vi "loadHTTemperature.vi"(8 "error in (no error)":errorcluster, 9 "Entity":string="QAMT03", 11 "file (use dialog)":path=path "C:/temp/ht/Temperature/temperatureLog.txt") -> (0 "error out":errorcluster)   [LabVIEW 2012]
uses:
  <vilib>/addons/database/Connection.llb/DB Tools Open Connec (Path).vi
  <vilib>/addons/database/Connection.llb/Conn Execute.vi
  <vilib>/addons/database/Recordset.llb/Rec Fetch Integer Data (R).vi
  <vilib>/addons/database/Recordset.llb/Rec Destroy - Connection.vi
  <vilib>/addons/database/NI_Database_API.lvlib
panel:
  in  "Cluster":T1
  out "before substring 2":string
  out "before substring":string
  out "date/time string":string
  out "text":string
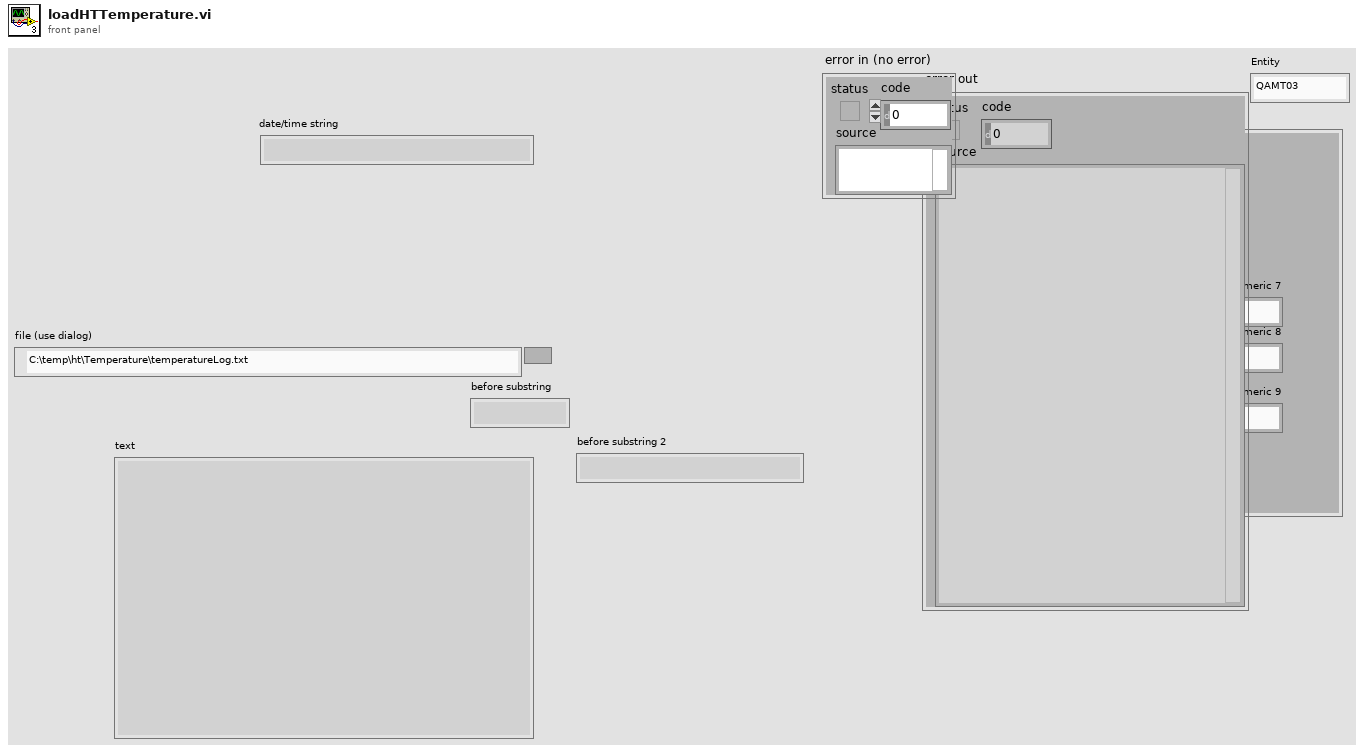
[diagram p1: front panel]
types:
  T1 = cluster{"Entity":string, "Time":string, "Numeric":dbl, "Numeric 2":dbl, "Numeric 3":dbl, "Numeric 4":dbl, "Numeric 5":dbl, "Numeric 6":dbl, "Numeric 7":dbl, "Numeric 8":dbl, "Numeric 9":dbl}
  T2 = typedef "NI_Database_API.lvlib/Conn ObjectReference.ctl" = refnum<k1>
  T3 = typedef "NI_Database_API.lvlib/Rec ObjectReference.ctl" = refnum<k1>
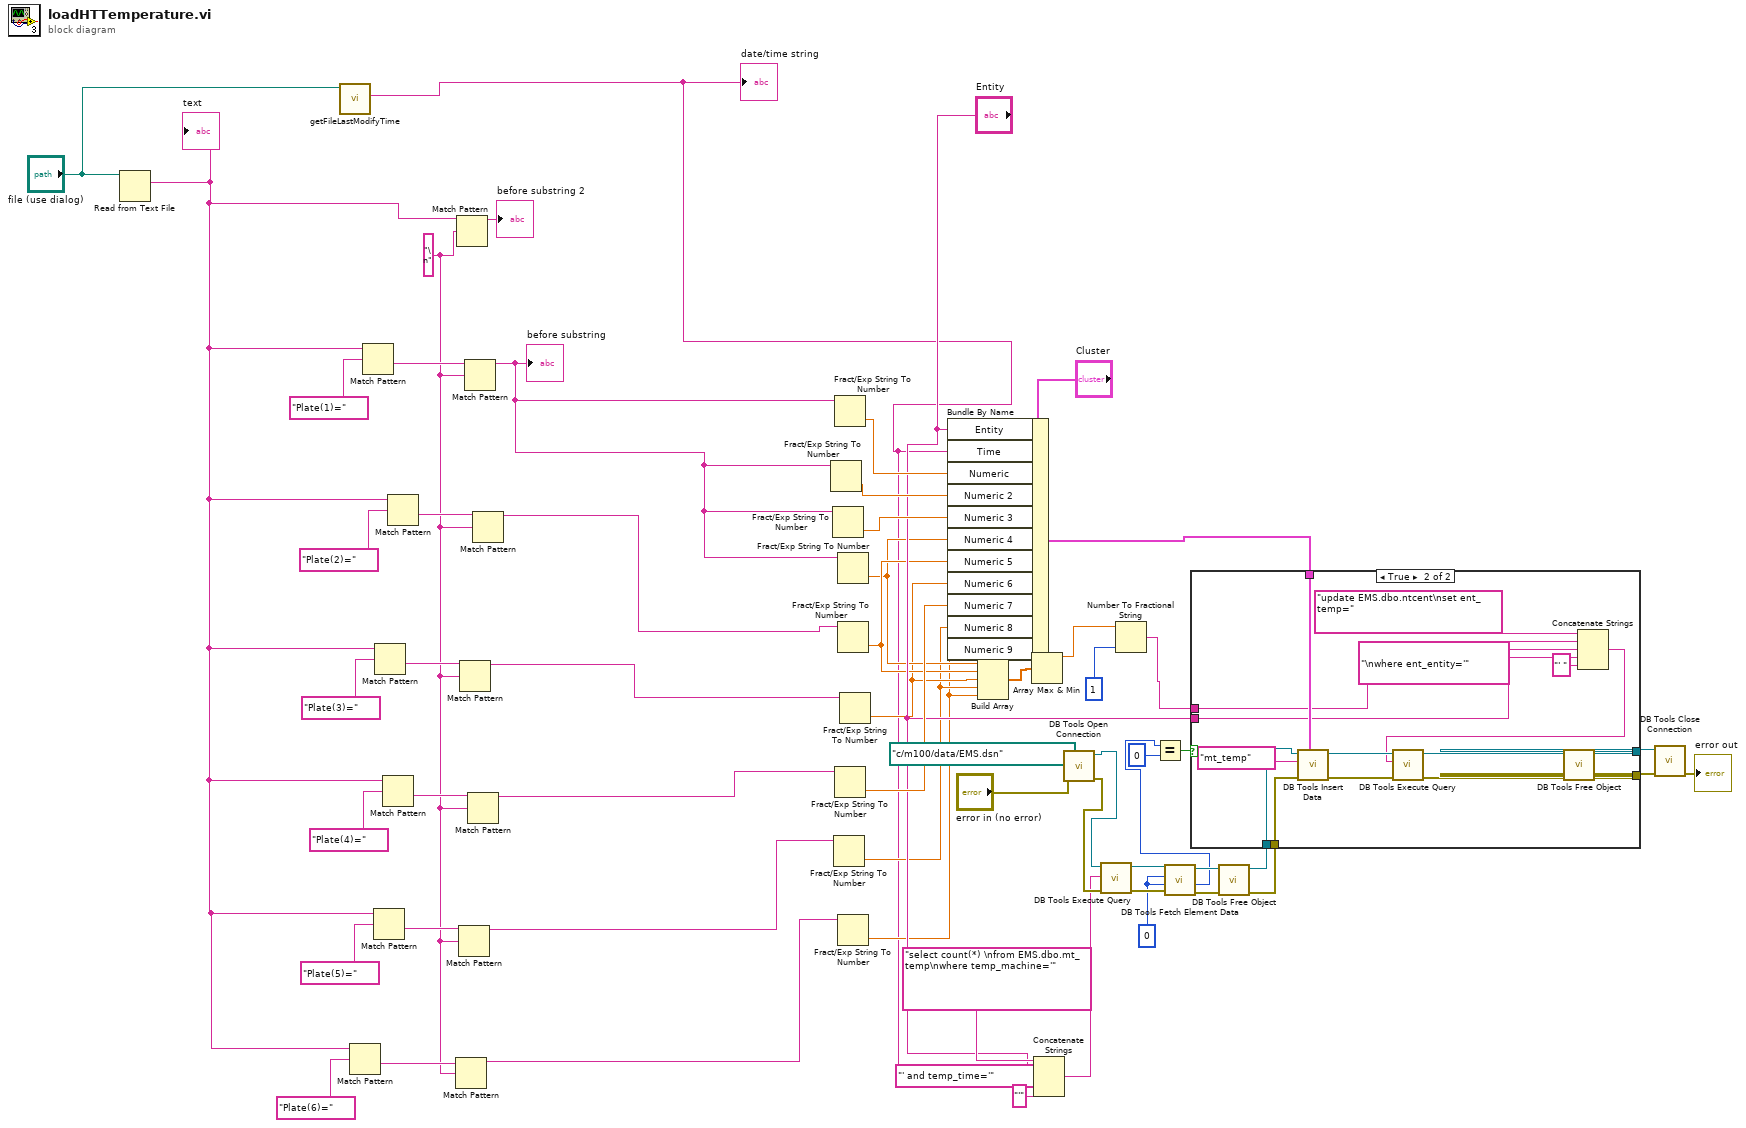
[diagram p0: block diagram]
diagram:
  w24 = 0
  w46 = "\n" ("regular expression")
  n1 = Read from Text File(file (use dialog)="file (use dialog)") -> (text=w47:string)  [unwired: 3 in, 3 out]
  "text" <- w47
  n2 = call "getFileLastModifyTime.vi"("path"="file (use dialog)") -> ("date/time string"=w7:string)  [unwired: 10 in]
  "date/time string" <- w7
  n3 = Match Pattern(string=w47, regular expression="Plate(6)=") -> (after substring=w49:string)  [unwired: 1 in, 3 out]
  n4 = Match Pattern(string=w47, regular expression="Plate(1)=") -> (after substring=w59:string)  [unwired: 1 in, 3 out]
  n5 = Match Pattern(string=w47, regular expression="Plate(5)=") -> (after substring=w51:string)  [unwired: 1 in, 3 out]
  n6 = Match Pattern(string=w47, regular expression="Plate(3)=") -> (after substring=w55:string)  [unwired: 1 in, 3 out]
  n7 = Match Pattern(string=w47, regular expression="Plate(4)=") -> (after substring=w53:string)  [unwired: 1 in, 3 out]
  n8 = Match Pattern(string=w47, regular expression="Plate(2)=") -> (after substring=w57:string)  [unwired: 1 in, 3 out]
  n9 = Match Pattern(string=w49, regular expression=w46) -> (before substring=w6:string)  [unwired: 1 in, 3 out]
  n10 = Match Pattern(string=w47, regular expression=w46) -> (before substring=→"before substring 2":string)  [unwired: 1 in, 3 out]
  n11 = Match Pattern(string=w51, regular expression=w46) -> (before substring=w5:string)  [unwired: 1 in, 3 out]
  n12 = Match Pattern(string=w55, regular expression=w46) -> (before substring=w3:string)  [unwired: 1 in, 3 out]
  n13 = Match Pattern(string=w59, regular expression=w46) -> (before substring=w1:string)  [unwired: 1 in, 3 out]
  "before substring" <- w1
  n14 = Match Pattern(string=w53, regular expression=w46) -> (before substring=w4:string)  [unwired: 1 in, 3 out]
  n15 = Match Pattern(string=w57, regular expression=w46) -> (before substring=w2:string)  [unwired: 1 in, 3 out]
  n16 = Fract/Exp String To Number(string=w1) -> (number=w43:dbl)  [unwired: 3 in, 1 out]
  n17 = Fract/Exp String To Number(string=w1) -> (number=w42:dbl)  [unwired: 3 in, 1 out]
  n18 = Fract/Exp String To Number(string=w5) -> (number=w11:dbl)  [unwired: 3 in, 1 out]
  n19 = Fract/Exp String To Number(string=w1) -> (number=w18:dbl)  [unwired: 3 in, 1 out]
  n20 = Fract/Exp String To Number(string=w4) -> (number=w41:dbl)  [unwired: 3 in, 1 out]
  n21 = Fract/Exp String To Number(string=w1) -> (number=w13:dbl)  [unwired: 3 in, 1 out]
  n22 = Fract/Exp String To Number(string=w2) -> (number=w14:dbl)  [unwired: 3 in, 1 out]
  n23 = Fract/Exp String To Number(string=w6) -> (number=w10:dbl)  [unwired: 3 in, 1 out]
  n24 = Fract/Exp String To Number(string=w3) -> (number=w12:dbl)  [unwired: 3 in, 1 out]
  n25 = Bundle By Name(cluster="Cluster", "Entity"="Entity", "Time"=w7, "Numeric"=w18, "Numeric 2"=w43, "Numeric 3"=w42, "Numeric 4"=w13, "Numeric 5"=w14, "Numeric 6"=w12, "Numeric 7"=w41, "Numeric 8"=w11, "Numeric 9"=w10) -> (w36:T1)
  n26 = Build Array(w13, w14, w12, w11, w10) -> (w9:dbl[])
  n27 = Array Max & Min(array=w9) -> (max value=w8:dbl)  [unwired: 3 out]
  n28 = Concatenate Strings("select count(*) \nfrom EMS.dbo.mt_temp\nwhere temp_machine='" ("string"), "Entity", "' and temp_time='" ("string"), w7, "'" ("string")) -> (w19:string)
  n29 = call-poly <vilib>:"DB Tools Open Connection.vi"("error in (no error)"="error in (no error)", "connection information"=path "c:/m100/data/EMS.dsn") -> ("error out"=w29:errorcluster, "connection reference"=w30:T2)  [unwired: 6 in]
  n30 = call-poly <vilib>:"DB Tools Execute Query.vi"("error in (no error)"=w29, "SQL query"=w19, "connection reference"=w30) -> ("error out"=w33:errorcluster, "recordset reference"=w32:T3)  [unwired: 5 in]
  n31 = Number To Fractional String(number=w8, precision (6)=i16 1 ("width (-)")) -> (F-format string=w16:string)  [unwired: 2 in]
  n32 = call-poly <vilib>:"DB Tools Fetch Element Data.vi"("error in (no error)"=w33, "type"=w24, "column index"=w24, "recordset reference"=w32) -> ("error out"=w34:errorcluster, "data"=w25:i32, "recordset reference out"=w31:T3)  [unwired: 3 in]
  n33 = Equal?(x=w25, y=0) -> (x = y?=w26:bool)
  n34 = call-poly <vilib>:"DB Tools Free Object.vi"("error in (no error)"=w34, "recordset reference"=w31) -> ("error out"=w27:errorcluster, "connection reference"=w28:T2)  [unwired: 8 in]
  n35 = case shown="True" w26 {
    tunnel: [w62 w73] -> w39
    tunnel: [w61 w71] -> w38
    tunnel: w36 -> [_ w77]
    tunnel: w28 -> [w62 w76]
    tunnel: w27 -> [w61 w75]
    tunnel: w16 -> [_ w67]
    tunnel: "Entity" -> [_ w65]
    frame False {
    }
    frame True {
      n36 = call <vilib>:"DB Tools Insert Data.vi"("data"=w77, "error in (no error)"=w75, "table"="mt_temp", "connection reference"=w76) -> ("error out"=w72:errorcluster, "connection reference out"=w74:T2)  [unwired: 6 in]
      n37 = Concatenate Strings("update EMS.dbo.ntcent\nset ent_temp=" ("string"), w67, "\nwhere ent_entity='" ("string"), w65, "' " ("string")) -> (w63:string)
      n38 = call-poly <vilib>:"DB Tools Execute Query.vi"("error in (no error)"=w72, "SQL query"=w63, "connection reference"=w74) -> ("error out"=w69:errorcluster, "recordset reference"=w70:T3)  [unwired: 5 in]
      n39 = call-poly <vilib>:"DB Tools Free Object.vi"("error in (no error)"=w69, "recordset reference"=w70) -> ("error out"=w71:errorcluster, "connection reference"=w73:T2)  [unwired: 8 in]
    }
  }
  n40 = call <vilib>:"DB Tools Close Connection.vi"("error in (no error)"=w38, "connection reference"=w39) -> ("error out"=→"error out":errorcluster)  [unwired: 5 in]
